vi "write_params.vi"(8 "error in (no error)":errorcluster caption="entrée d'erreur (pas d'erreur)", 10 "params":T1={"fit_intercept"=TRUE, "normalize"=FALSE, "copy_X"=TRUE, "n_jobs"=1.0, "positive"=FALSE}, 11 "LinearRegression en entrée":refnum<class "LinearRegression.lvclass">) -> (0 "error out":errorcluster caption="sortie d'erreur", 3 "LinearRegression en sortie":refnum<class "LinearRegression.lvclass">)   [LabVIEW 2020, in "LinearRegression.lvclass"]
uses:
  LinearRegression.lvclass
  Controls/linear_regression_params.ctl
  LinearRegression.lvclass/LinearRegression.ctl
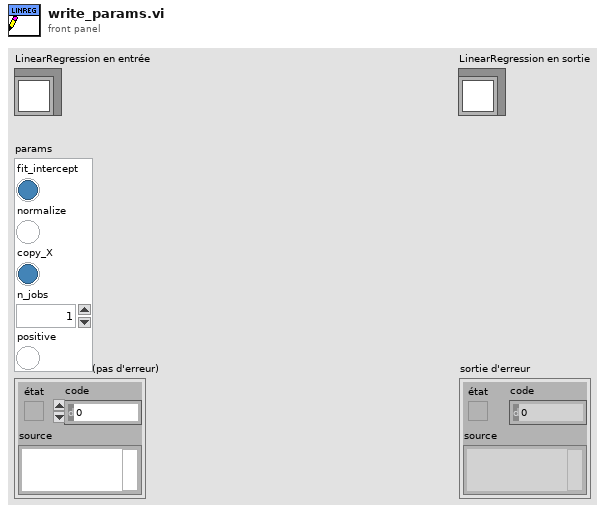
[diagram p1: front panel]
types:
  T1 = typedef "linear_regression_params.ctl" = cluster{"fit_intercept":bool, "normalize":bool, "copy_X":bool, "n_jobs":dbl, "positive":bool}
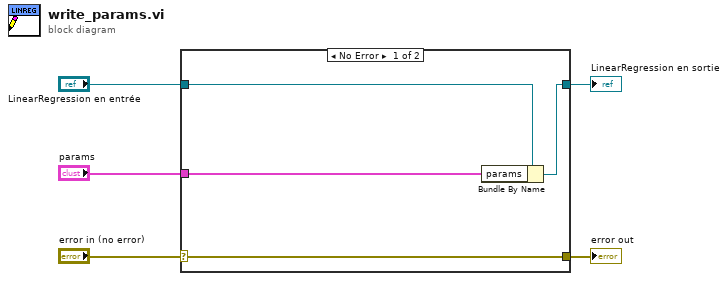
[diagram p0: block diagram]
diagram:
  n1 = case shown="No Error" "error in (no error)" {
    selector: "error in (no error)" -> [w9 w10]
    tunnel: [w9 w10] -> w4
    tunnel: [w7 w11] -> w2
    tunnel: "LinearRegression en entrée" -> [w8 w11]
    tunnel: "params" -> [w6 _]
    frame No Error {
      n2 = Bundle By Name(cluster=w8, "params"=w6) -> (w7:refnum<class "LinearRegression.lvclass">)
    }
    frame Error {
    }
  }
  "error out" <- w4
  "LinearRegression en sortie" <- w2
